vi "Module Type.vi"(11 "Role Manager in":refnum<class "Role Manager.lvclass">) -> (2 "Module Type":string)   [LabVIEW 2020, in "Volatus.lvlib" / "Role Manager.lvclass"]
uses:
  Role Manager.lvclass
  Role Manager.lvclass/Role Manager.ctl
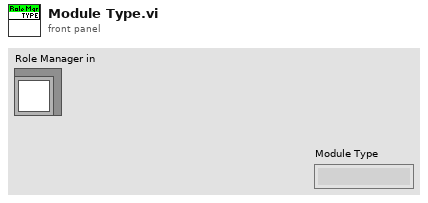
[diagram p1: front panel]
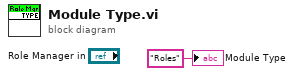
[diagram p0: block diagram]
diagram:
  "Module Type" <- "Roles" ("Module Type")
